vi "FTW-ProjectItemManager-Delete.vi"(0 "Project Item Manager":refnum<class "FTW-ProjectItemManager.lvclass">, 5 "Regex Matches to Delete":string, 11 "error in":errorcluster) -> (4 "Project Item Manager out":refnum<class "FTW-ProjectItemManager.lvclass">, 15 "error out":errorcluster)   [LabVIEW 2012, in "FTW-ProjectItemManager.lvclass"]
uses:
  FTW-ProjectItemManager.lvclass
  FTW-ProjectItemManager.lvclass/FTW-ProjectItemManager.ctl
panel:
  out "Tags Deleted":string[](array[string])
  # "Inputs"
  # "Outputs"
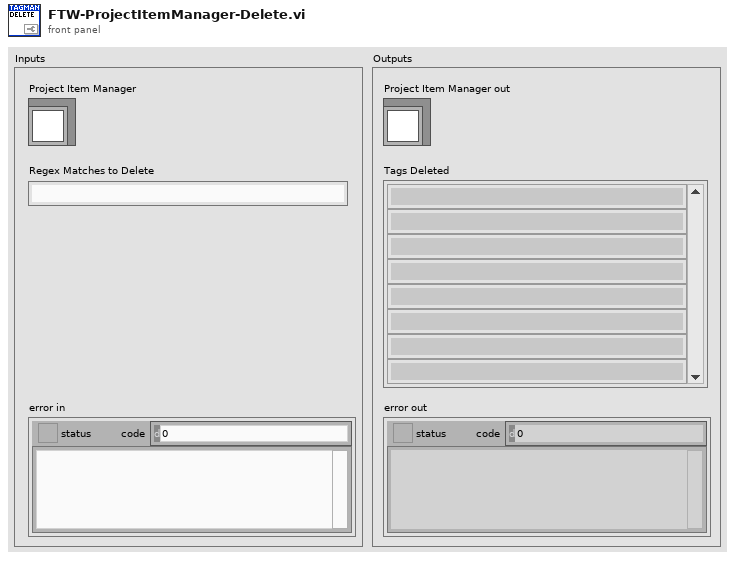
[diagram p1: front panel]
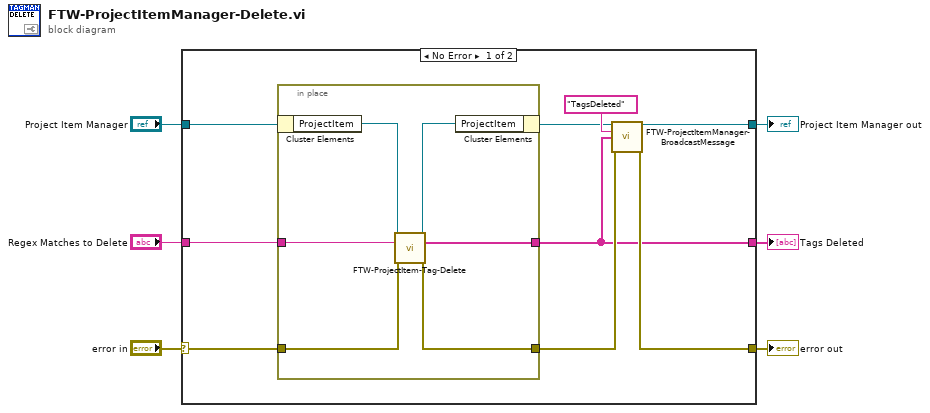
[diagram p0: block diagram]
diagram:
  n1 = case shown="No Error" "error in" {
    selector: "error in" -> [w15 w23]
    tunnel: [w13 w23] -> w6
    tunnel: [w14 w22] -> w4
    tunnel: "Project Item Manager" -> [w8 w22]
    tunnel: "Regex Matches to Delete" -> [w10 _]
    tunnel: [w9 _] -> w1
    frame No Error {
      n2 = in-place {
        in-place-border: w15 -> [w21]
        in-place-border: [w20] -> w12
        in-place-border: w10 -> [w19]
        in-place-border: [w18] -> w9
        n3 = in-place-cluster #1(w8) -> ("ProjectItem"=w17:refnum<vi>)
        n4 = call "FTW-ProjectItem-Tag-Delete.vi"("ProjectItem"=w17, "Tag Name Regex Matches to Delete"=w19, "error in"=w21) -> ("ProjectItem out"=w16:refnum<vi>, "Tags Deleted"=w18:string[], "error out"=w20:errorcluster)  [unwired: 10 in]
        n5 = in-place-cluster #1("ProjectItem"=w16) -> (w7:refnum<class "FTW-ProjectItemManager.lvclass">)
      }
      n6 = call "FTW-ProjectItemManager-BroadcastMessage.vi"("Project Item Manager"=w7, "Action Performed"="TagsDeleted", "Payload"=w9, "error in"=w12) -> ("Project Item Manager out"=w14:refnum<class "FTW-ProjectItemManager.lvclass">, "error out"=w13:errorcluster)  [unwired: 10 in]
    }
    frame Error {
    }
  }
  "error out" <- w6
  "Project Item Manager out" <- w4
  "Tags Deleted" <- w1
